vi "Plot Contours.vi"(8 "error in (no error)":errorcluster, 9 "Color":u32(colorbox)=16711680, 10 "Boundaries":T1(array[cluster]), 11 "Image In":T2) -> (0 "error out":errorcluster, 3 "Image":T2(plugin-control))   [LabVIEW 2012, in "Visual Analyser.lvlib"]
uses:
  Visual Analyser.lvlib
  <vilib>/vision/Image Controls.llb/IMAQ Image.ctl
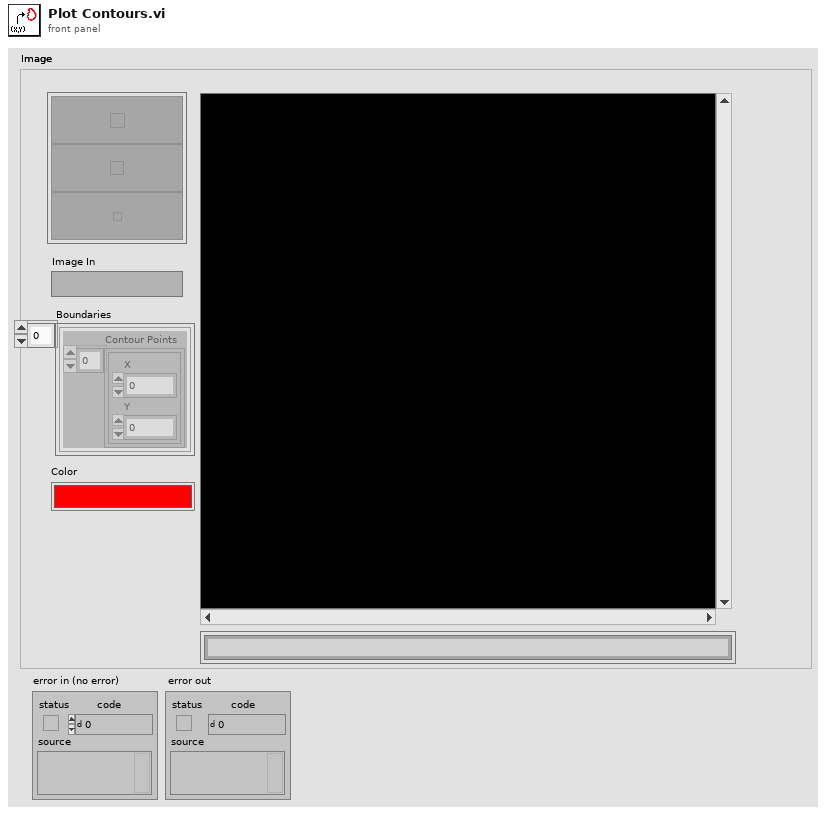
[diagram p1: front panel]
types:
  T1 = cluster{"Contour Points":cluster{"X":i32, "Y":i32}[]}[]
  T2 = typedef "IMAQ Image.ctl" = refnum<image>
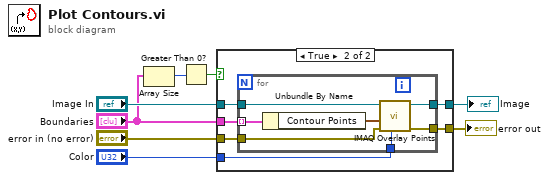
[diagram p0: block diagram]
diagram:
  n1 = Array Size(array="Boundaries") -> (size(s)=w2:i32)
  n2 = Greater Than 0?(x=w2) -> (x > 0?=w1:bool)
  n3 = case shown="True" w1 {
    tunnel: [w10 w16] -> w8
    tunnel: "Color" -> [_ w15]
    tunnel: "Image In" -> [w10 w14]
    tunnel: "Boundaries" -> [_ w13]
    tunnel: "error in (no error)" -> [w9 w12]
    tunnel: [w9 w11] -> w4
    frame False {
    }
    frame True {
      n4 = for {
        tunnel: w13 -> [w21] mode=indexing
        tunnel: [w23] -> w16
        tunnel: w15 -> [w20]
        tunnel: w14 -> [w19]
        tunnel: w12 -> [w18]
        tunnel: [w17] -> w11
        n5 = Unbundle By Name(w21) -> ("Contour Points"=w22:cluster{"X":i32, "Y":i32}[])
        n6 = call "IMAQ Overlay Points"("Color"=w20, "error in (no error)"=w18, "Array of Points"=w22, "Image"=w19) -> ("error out"=w17:errorcluster, "Image Out"=w23:T2)  [unwired: 6 in]
      }
    }
  }
  "Image" <- w8
  "error out" <- w4
